vi "Update Status Channels.vi"(4 "Finished Late? [i-1]":bool, 6 "Iteration Duration":i64, 8 "error in (no error)":errorcluster, 11 "Status Group Reference":T1) -> (0 "error out":errorcluster)   [LabVIEW 2017, in "NI 272x Resistive Simulation Custom Device Engine.lvlib"]
uses:
  NI 272x Resistive Simulation Custom Device Engine.lvlib
  <vilib>/NI/NIVS Inline Async API/_Data Access Engine/Data Access Engine/Types/Write.DVR.ctl
  <vilib>/NI/NIVS Inline Async API/_Data Access Engine/Access Type Classes/Write/Write.lvclass
  <vilib>/NI/NIVS Inline Async API/_Data Access Engine/Access Type Classes/Write/Write.lvclass/Write.ctl
  <vilib>/NI/NIVS Inline Async API/_Data Access Engine/Data Access Engine/Methods/Write.Data.vi
  <vilib>/NI/NIVS Inline Async API/_Data Access Engine/Access Type Classes/Write/Write.ProcessData.vi
  <vilib>/NI/NIVS Inline Async API/_Data Access Engine/Data Access Engine/Data Access Engine.lvclass
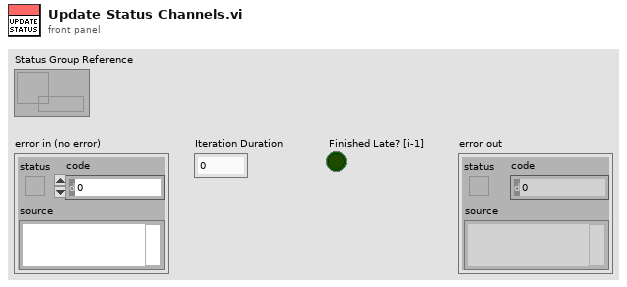
[diagram p1: front panel]
types:
  T1 = typedef "Data Access Engine.lvlib/Data Access Engine.lvclass/Write.DVR.ctl" = refnum<data-value>
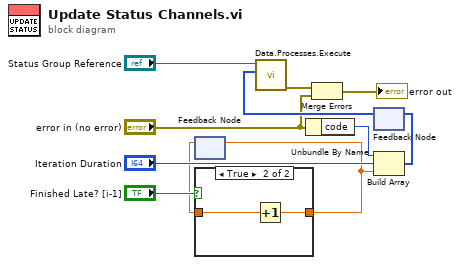
[diagram p0: block diagram]
diagram:
  n1 = feedback #1() -> (w8:dbl)  [unwired: 1 in]
  n2 = case shown="True" "Finished Late? [i-1]" {
    tunnel: w8 -> [w12 w13]
    tunnel: [w12 w14] -> w7
    frame False {
    }
    frame True {
      n3 = Increment(x=w13) -> (x+1=w14:dbl)
    }
  }
  n4 = feedback-in #1(w7) -> ()
  n5 = Unbundle By Name("error in (no error)") -> ("code"=w6:i32)
  n6 = feedback #2() -> (w4:i64[])  [unwired: 1 in]
  n7 = call-poly <vilib>:"Data.Processes.Execute.vi"("Values"=w4, "Ref"="Status Group Reference") -> ("error out"=w3:errorcluster)  [unwired: 9 in]
  n8 = Merge Errors(w3, "error in (no error)") -> (→"error out":errorcluster)
  n9 = Build Array(w6, "Iteration Duration", w7) -> (w5:i64[])
  n10 = feedback-in #2(w5) -> ()
